vi "Write U32.vi"(8 "error in (no error)":errorcluster, 9 "Default If Not Found":u32, 10 "Name":string, 11 "IConfiguration in":refnum<class "IConfiguration.lvclass">) -> (0 "error out":errorcluster, 3 "IConfiguration out":refnum<class "IConfiguration.lvclass">)   [LabVIEW 2017, in "Configuration.lvlib" / "IConfiguration.lvclass"]
uses:
  IConfiguration.lvclass
  <vilib>/Utility/Data Type/Type Definitions/Data Type.ctl
  <vilib>/Utility/Data Type/NI_Data Type.lvlib
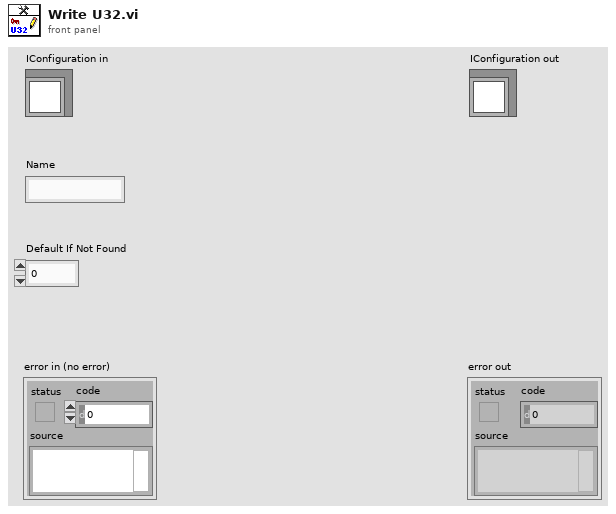
[diagram p1: front panel]
types:
  T1 = typedef "NI_Data Type.lvlib/Data Type.ctl" = enum8{"Invalid Type", "Void", "I8", "I16", "I32", "I64", "U8", "U16", "U32", "U64", "Single Float", "Double Float", "Extended Float", "Single Complex", "Double Complex", "Extended Complex", "Enum U8", "Enum U16", "Enum U32", "Enum U64", "Single Float With Unit", "Double Float With Unit", "Extended Float With Unit", "Single Complex with Unit", "Double Complex with Unit", "Extended Complex with Unit", "Boolean", "String", "Path", "Picture", "Tag", "Array", "Cluster", "Variant", "LV Variant", "Waveform", "Timestamp", "Digital Waveform", "Digital Data", "ExpressData", "Refnum", "External Data", "VI", "Poly VI", "LabVIEW Class Instance", "Fixed Point"}
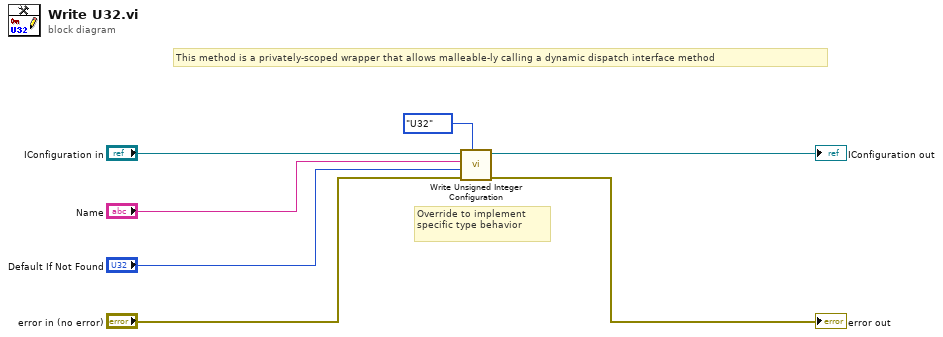
[diagram p0: block diagram]
diagram:
  # "Override to implement\nspecific type behavior"
  # "This method is a privately-scoped wrapper that allows malleable-ly calling a dynamic dispatch interface method"
  n1 = call-dynamic "Write Unsigned Integer Configuration.vi"("Type"=Data_Type."U32", "error in (no error)"="error in (no error)", "Value"="Default If Not Found", "Name"="Name", "IConfiguration in"="IConfiguration in") -> ("error out"=→"error out":errorcluster, "IConfiguration out"=→"IConfiguration out":refnum<class "IConfiguration.lvclass">)  [unwired: 5 in]
